vi "byte_array_to_bool_array_teardown.vi"(8 "error in (no error)":errorcluster, 10 "Array":bool[](array[boolean])) -> (0 "error out":errorcluster, 1 "32nd bit":bool, 2 "0th bit":bool)   [LabVIEW 2018]
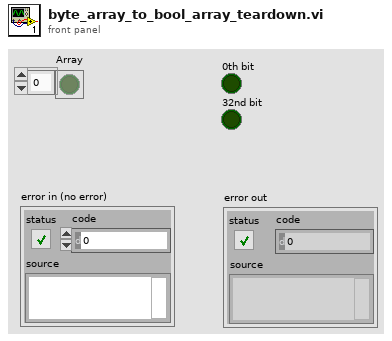
[diagram p1: front panel]
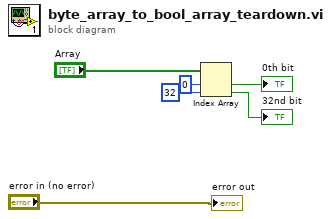
[diagram p0: block diagram]
diagram:
  n1 = Index Array(array="Array", index #1=0 ("index"), index #2=32 ("index")) -> (element #1=→"0th bit":bool, element #2=→"32nd bit":bool)
  "error out" <- "error in (no error)"
